vi "Read Loop.vi"(8 "error in (no error)":errorcluster, 11 "WAMP Client in":refnum<class "WAMP Client.lvclass">) -> (0 "error out":errorcluster, 3 "WAMP Client out":refnum<class "WAMP Client.lvclass">)   [LabVIEW 2020, in "wamplv.lvlib" / "WAMP Client.lvclass"]
uses:
  <userlib>/wamplv/WAMP Client/WAMP Client.lvclass
  <userlib>/wamplv/WAMP Client/WAMP Client.lvclass/WAMP Client.ctl
  <userlib>/wamplv/WAMP Client/TypeDef/Internal Message.ctl
  <userlib>/wamplv/WAMP Client/TypeDef/Internal Message Type.ctl
  <userlib>/wamplv/WAMP Client/TypeDef/Termination Reason Enum.ctl
  <vilib>/JDP Science/JSONtext/Get Array Elements.vi
  <vilib>/Utility/error.llb/Error Cluster From Error Code.vi
  <vilib>/ErrorRing/Error Ring.xnode
  <userlib>/wamplv/Comm Handlers/ICommHandler/ICommHandler.lvclass
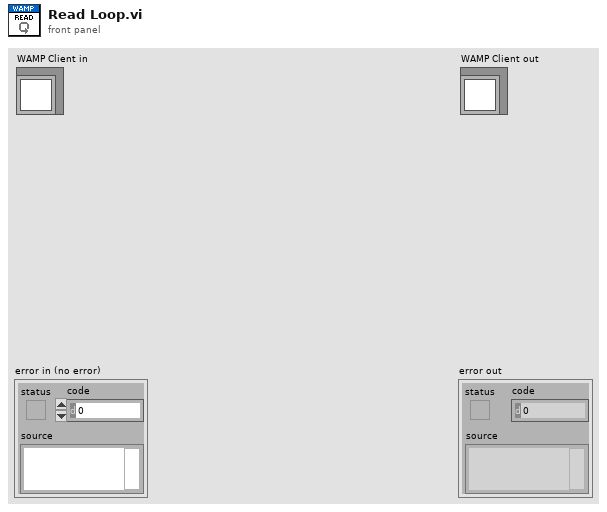
[diagram p1: front panel]
types:
  T1 = typedef "wamplv.lvlib/WAMP Client.lvclass/Termination Reason Enum.ctl" = enum16{"Goodbye Received", "Abort Received", "Send Goodbye", "Send Abort", "Read Loop Failure", "Write Loop Failure", "Message Loop Failure"}
  T2 = typedef "wamplv.lvlib/WAMP Client.lvclass/Internal Message Type.ctl" = enum16{"Subscribe", "Handle Subscribed", "Handle Event", "Unsubscribe", "Handle Unsubscribed", "Publish", "Handled Published", "Goodbye", "Handle Goodbye", "Call", "Handle Result", "Register", "Handle Registered", "Unregister", "Handle Unregistered", "Handle Invocation", "Yield", "Error"}
  T3 = typedef "wamplv.lvlib/WAMP Client.lvclass/Internal Message.ctl" = cluster{"Internal Message Type":T2, "Variant":variant}
  T4 = typedef "wamplv.lvlib/WAMP Client.lvclass/WAMP Message Codes.ctl" = u16
  T5 = typedef "wamplv.lvlib/WAMP Client.lvclass/WAMP Received Message.ctl" = cluster{"Message JSON":string[], "Message Codes":T4}
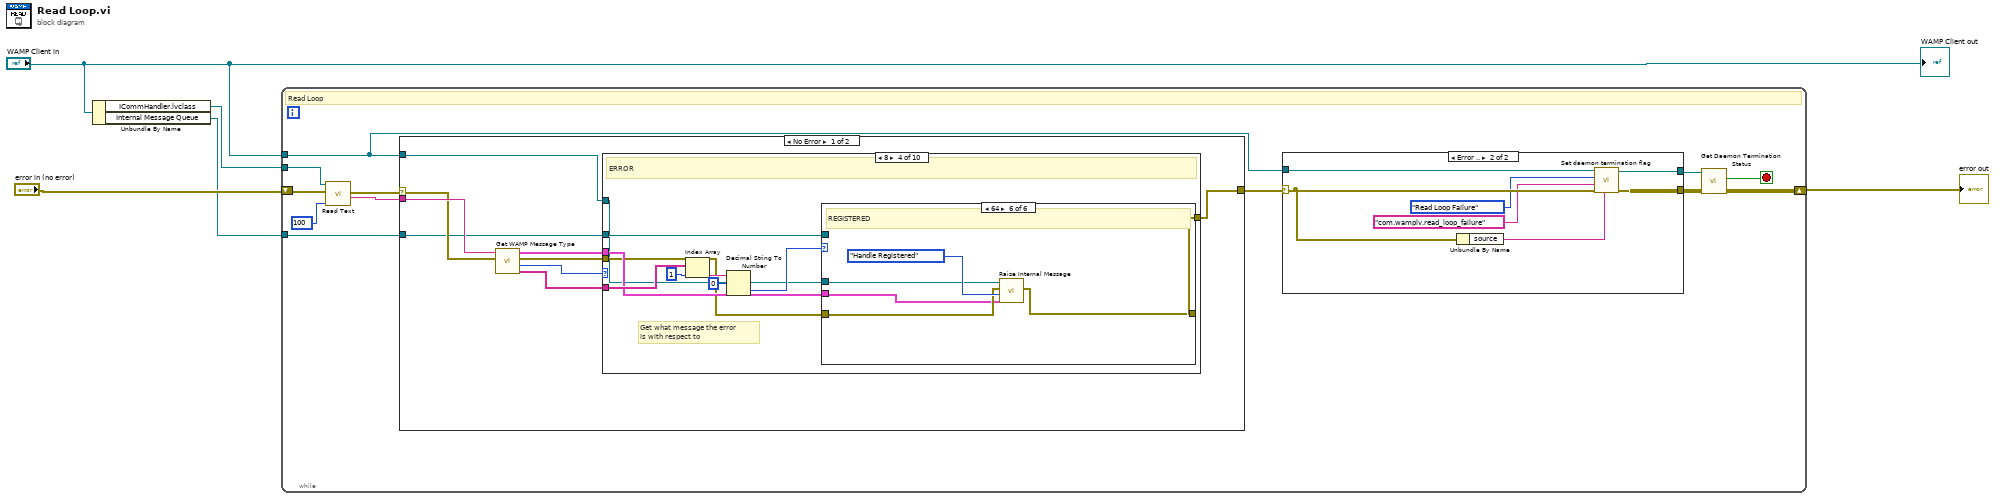
[diagram p0: block diagram]
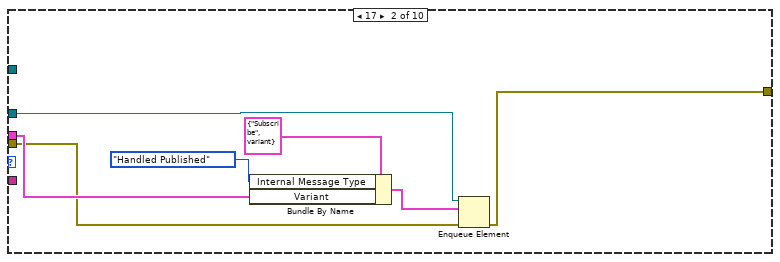
[diagram p4: hidden frame]
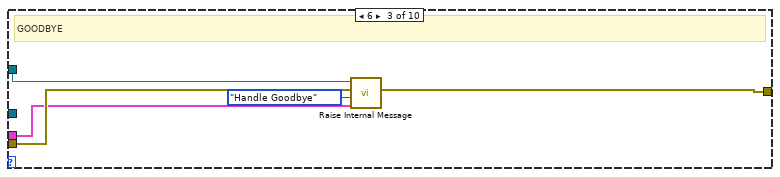
[diagram p5: hidden frame]
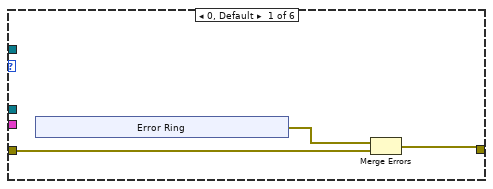
[diagram p6: hidden frame]
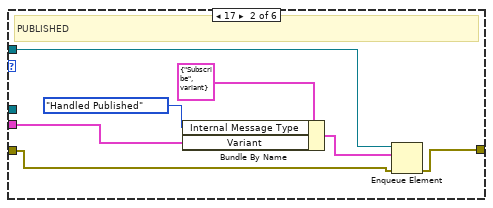
[diagram p7: hidden frame]
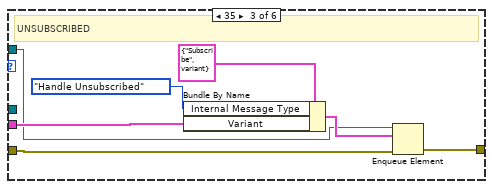
[diagram p8: hidden frame]
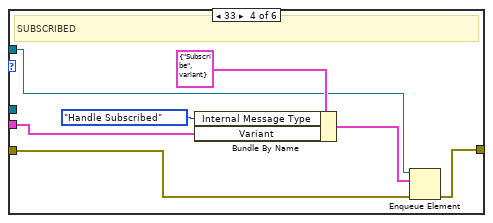
[diagram p9: hidden frame]
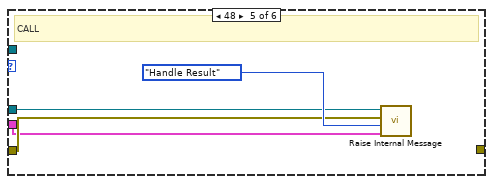
[diagram p10: hidden frame]
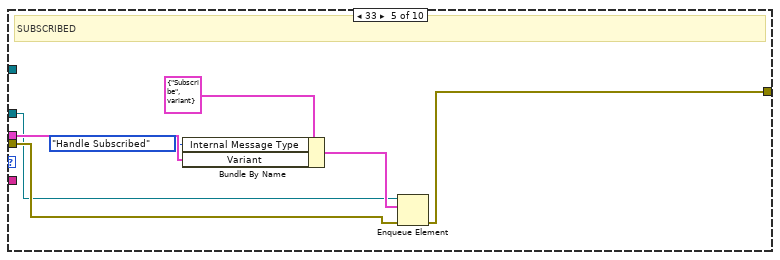
[diagram p11: hidden frame]
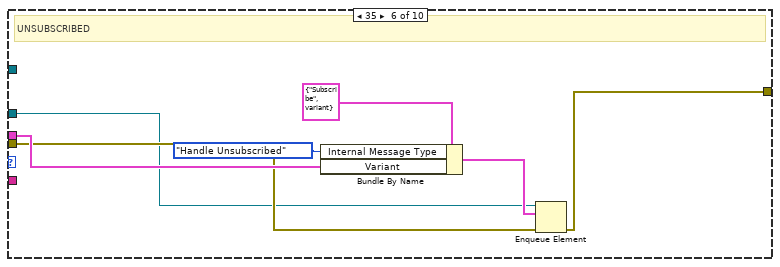
[diagram p12: hidden frame]
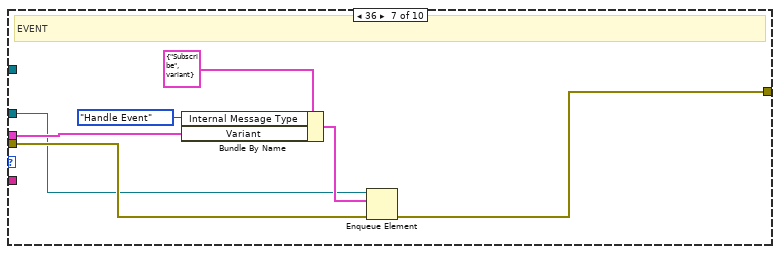
[diagram p13: hidden frame]
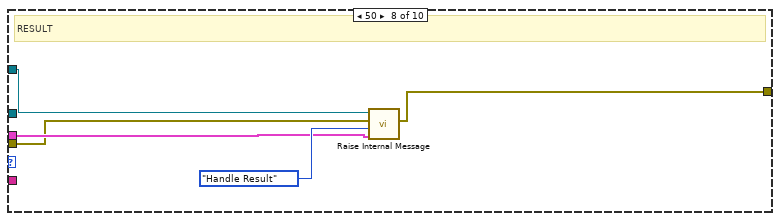
[diagram p14: hidden frame]
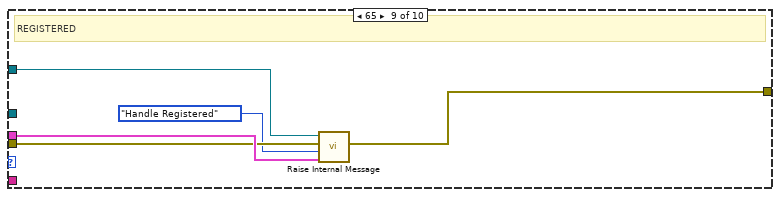
[diagram p15: hidden frame]
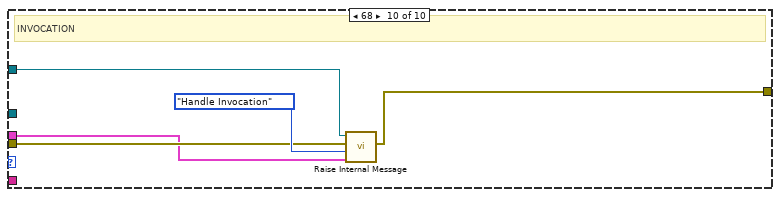
[diagram p16: hidden frame]
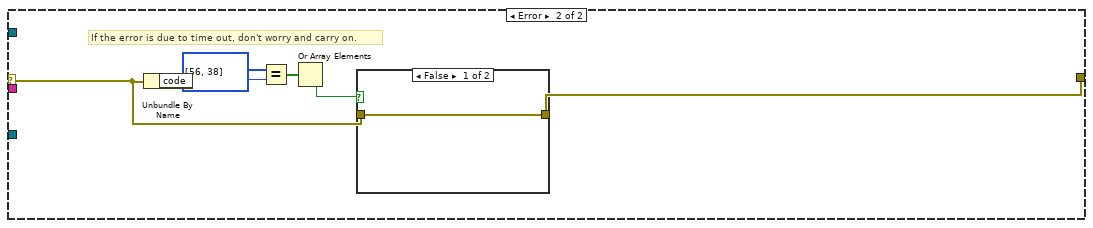
[diagram p17: hidden frame]
diagram:
  n1 = Unbundle By Name("WAMP Client in") -> ("ICommHandler.lvclass"=w4:refnum<class "ICommHandler.lvclass">, "Internal Message Queue"=w2:refnum<queue>)
  n2 = while {
    shift-right: [w7] -> w3
    shift-left: "error in (no error)" -> [w17]
    tunnel: w4 -> [w13]
    tunnel: w2 -> [w12]
    tunnel: "WAMP Client in" -> [w6]
    stop <- w8 stop-if-true
    # "Read Loop"
    n3 = call-dynamic "Read Text.vi"("timeout ms (5000)"=100, "error in (no error)"=w17, "ICommHandler in"=w13) -> ("String"=w14:string, "error out"=w15:errorcluster)  [unwired: 4 in, 1 out]
    n4 = case shown="No Error" w15 {
      selector: w15 -> [w30 w138]
      tunnel: [w29 w137] -> w11
      tunnel: w14 -> [w31 _]
      tunnel: w12 -> [w28 _]
      tunnel: w6 -> [w27 _]
      frame No Error {
        n5 = call <userlib>:"Get WAMP Message Type.vi"("error in (no error)"=w30, "JSON"=w31) -> ("<JSON>"=w33:string[], "Message Codes"=w32:T4, "error out"=w34:errorcluster, "WAMP Message"=w35:T5)  [unwired: 6 in]
        n6 = case shown="8" w32 {
          tunnel: w33 -> [_ _ _ w55 _ _ _ _ _ _]
          tunnel: w34 -> [w36 w39 w47 w53 w99 w106 w114 w120 w125 w130]
          tunnel: w35 -> [_ w40 w45 w54 w101 w108 w115 w121 w126 w128]
          tunnel: [w36 w38 w44 w52 w100 w107 w113 w119 w124 w129] -> w29
          tunnel: w28 -> [_ w37 _ w50 w97 w104 w111 _ _ _]
          tunnel: w27 -> [_ _ w48 w49 _ _ _ w118 w127 w132]
          frame 0, Default {
          }
          frame 17 {
            n7 = Bundle By Name(cluster=T3 {"Internal Message Type"=enum."Subscribe", "Variant"=variant} ("Cluster"), "Internal Message Type"=Internal_Message_Type."Handled Published", "Variant"=w40) -> (w42:T3)
            n8 = Enqueue Element(queue=w37, element=w42, error in (no error)=w39) -> (error out=w38:errorcluster)  [unwired: 1 in, 2 out]
          }
          frame 6 {
            # "GOODBYE"
            n9 = call-dynamic "Raise Internal Message.vi"("Variant"=w45, "Internal Message Type"=Internal_Message_Type."Handle Goodbye", "error in (no error)"=w47, "WAMP Client in"=w48) -> ("error out"=w44:errorcluster)  [unwired: 6 in, 1 out]
          }
          frame 8 {
            # "Get what message the error \nis with respect to"
            # "ERROR"
            n10 = Index Array(array=w55, index=1) -> (element=w57:string)
            n11 = Decimal String To Number(string=w57, offset=0) -> (number=w56:i32)  [unwired: 1 in, 1 out]
            n12 = case shown="64" w56 {
              tunnel: w54 -> [_ w69 w77 w85 w89 w92]
              tunnel: w53 -> [w60 w70 w76 w84 w90 w94]
              tunnel: [w61 w68 w75 w83 _ w93] -> w52
              tunnel: w50 -> [_ w67 w74 w81 _ _]
              tunnel: w49 -> [_ _ _ _ w88 w95]
              frame 0, Default {
                n13 = xnode "Error Ring"() -> ("error out"=w59:errorcluster)
                n14 = Merge Errors(w59, w60) -> (w61:errorcluster)
              }
              frame 17 {
                # "PUBLISHED"
                n15 = Bundle By Name(cluster=T3 {"Internal Message Type"=enum."Subscribe", "Variant"=variant} ("Cluster"), "Internal Message Type"=Internal_Message_Type."Handled Published", "Variant"=w69) -> (w72:T3)
                n16 = Enqueue Element(queue=w67, element=w72, error in (no error)=w70) -> (error out=w68:errorcluster)  [unwired: 1 in, 2 out]
              }
              frame 35 {
                # "UNSUBSCRIBED"
                n17 = Bundle By Name(cluster=T3 {"Internal Message Type"=enum."Subscribe", "Variant"=variant} ("Cluster"), "Internal Message Type"=Internal_Message_Type."Handle Unsubscribed", "Variant"=w77) -> (w79:T3)
                n18 = Enqueue Element(queue=w74, element=w79, error in (no error)=w76) -> (error out=w75:errorcluster)  [unwired: 1 in, 2 out]
              }
              frame 33 {
                # "SUBSCRIBED"
                n19 = Bundle By Name(cluster=T3 {"Internal Message Type"=enum."Subscribe", "Variant"=variant} ("Cluster"), "Internal Message Type"=Internal_Message_Type."Handle Subscribed", "Variant"=w85) -> (w86:T3)
                n20 = Enqueue Element(queue=w81, element=w86, error in (no error)=w84) -> (error out=w83:errorcluster)  [unwired: 1 in, 2 out]
              }
              frame 48 {
                # "CALL"
                n21 = call-dynamic "Raise Internal Message.vi"("Variant"=w89, "Internal Message Type"=Internal_Message_Type."Handle Result", "error in (no error)"=w90, "WAMP Client in"=w88) -> ()  [unwired: 6 in, 2 out]
              }
              frame 64 {
                # "REGISTERED"
                n22 = call-dynamic "Raise Internal Message.vi"("Variant"=w92, "Internal Message Type"=Internal_Message_Type."Handle Registered", "error in (no error)"=w94, "WAMP Client in"=w95) -> ("error out"=w93:errorcluster)  [unwired: 6 in, 1 out]
              }
            }
          }
          frame 33 {
            # "SUBSCRIBED"
            n23 = Bundle By Name(cluster=T3 {"Internal Message Type"=enum."Subscribe", "Variant"=variant} ("Cluster"), "Internal Message Type"=Internal_Message_Type."Handle Subscribed", "Variant"=w101) -> (w102:T3)
            n24 = Enqueue Element(queue=w97, element=w102, error in (no error)=w99) -> (error out=w100:errorcluster)  [unwired: 1 in, 2 out]
          }
          frame 35 {
            # "UNSUBSCRIBED"
            n25 = Bundle By Name(cluster=T3 {"Internal Message Type"=enum."Subscribe", "Variant"=variant} ("Cluster"), "Internal Message Type"=Internal_Message_Type."Handle Unsubscribed", "Variant"=w108) -> (w109:T3)
            n26 = Enqueue Element(queue=w104, element=w109, error in (no error)=w106) -> (error out=w107:errorcluster)  [unwired: 1 in, 2 out]
          }
          frame 36 {
            # "EVENT"
            n27 = Bundle By Name(cluster=T3 {"Internal Message Type"=enum."Subscribe", "Variant"=variant} ("Cluster"), "Internal Message Type"=Internal_Message_Type."Handle Event", "Variant"=w115) -> (w116:T3)
            n28 = Enqueue Element(queue=w111, element=w116, error in (no error)=w114) -> (error out=w113:errorcluster)  [unwired: 1 in, 2 out]
          }
          frame 50 {
            # "RESULT"
            n29 = call-dynamic "Raise Internal Message.vi"("Variant"=w121, "Internal Message Type"=Internal_Message_Type."Handle Result", "error in (no error)"=w120, "WAMP Client in"=w118) -> ("error out"=w119:errorcluster)  [unwired: 6 in, 1 out]
          }
          frame 65 {
            # "REGISTERED"
            n30 = call-dynamic "Raise Internal Message.vi"("Variant"=w126, "Internal Message Type"=Internal_Message_Type."Handle Registered", "error in (no error)"=w125, "WAMP Client in"=w127) -> ("error out"=w124:errorcluster)  [unwired: 6 in, 1 out]
          }
          frame 68 {
            # "INVOCATION"
            n31 = call-dynamic "Raise Internal Message.vi"("Variant"=w128, "Internal Message Type"=Internal_Message_Type."Handle Invocation", "error in (no error)"=w130, "WAMP Client in"=w132) -> ("error out"=w129:errorcluster)  [unwired: 6 in, 1 out]
          }
        }
      }
      frame Error {
        # "If the error is due to time out, don't worry and carry on."
        n32 = Unbundle By Name(w138) -> ("code"=w136:i32)
        n33 = Equal?(x=i32[] [56, 38] ("y"), y=w136) -> (x = y?=w134:bool[])
        n34 = Or Array Elements(Boolean array=w134) -> (logical OR=w133:bool)
        n35 = case shown="False" w133 {
          tunnel: w138 -> [w139 _]
          tunnel: [w139 _] -> w137
          frame False {
          }
          frame True {
          }
        }
      }
    }
    n36 = case shown="Error .." w11 {
      selector: w11 -> [w19 w24]
      tunnel: [w19 w25] -> w9
      tunnel: [w18 w26] -> w10
      tunnel: w6 -> [w18 w23]
      frame No Error {
      }
      frame Error {
        n37 = Unbundle By Name(w24) -> ("source"=w21:string)
        n38 = call <userlib>:"Set daemon termination flag.vi"("Message"=w21, "error in (no error)"=w24, "Reason URI"="com.wamplv.read_loop_failure", "Reason"=Termination_Reason_Enum."Read Loop Failure" ("Termination Reason"), "WAMP Client (in)"=w23) -> ("error out"=w25:errorcluster, "WAMP Client (out)"=w26:refnum<class "WAMP Client.lvclass">)  [unwired: 5 in]
      }
    }
    n39 = call <userlib>:"Get Daemon Termination Status.vi"("error in (no error)"=w9, "WAMP Client in"=w10) -> ("error out"=w7:errorcluster, "Terminate?"=w8:bool)  [unwired: 6 in, 2 out]
  }
  "error out" <- w3
  "WAMP Client out" <- "WAMP Client in"
